vi "PB-01 Interface.vi"(6 "Device Inputs":dbl[](array[numeric]), 8 "error in":errorcluster, 9 "Device Outputs in":dbl[](array[numeric]), 10 "DCM Ref":refnum<class "DCM - RT.lvclass">, 11 "PB-01 in":T1={"FIFO Indexes"={"Write"={"Clear Faults"=0, "ESTTL Setup"=[], "UEGO Control"={"UEGO1Enable"=-1, "UEGO2Enable"=-1, "UEGO1Range"=-1, "UEGO2Range"=-1, "FilterCutoff (Hz)"=-1}}, "Read"={"UEGO Sensor Results"={"UEGO1Lambda"=-1, "UEGO1Phi"=-1, "UEGO1AFRatio"=-1, "UEGO1Ip (mA)"=-1, "UEGO2Lambda"=-1, "UEGO2Phi"=-1, "UEGO2AFRatio"=-1, "UEGO2Ip (mA)"=-1}, "UEGO Temperature (C)"={"UEGO1Temp (C)"=-1, "UEGO2Temp (C)"=-1, "UEGO1Hot"=-1, "UEGO2Hot"=-1}, "UEGO Diagnostics"={"UEGO1SensorFault"=-1, "UEGO2SensorFault"=-1, "UEGO1HeaterFault"=-1, "UEGO2HeaterFault"=-1, "UEGOFuseStatus"=-1, "Battery (V)"=-1, "LSUType"=-1}}}, "Settings"={"VR-Hall Mode Select"=[enum."VR Adaptive Arm", enum."VR Adaptive Arm", enum."VR Adaptive Arm", enum."VR Adaptive Arm", enum."VR Adaptive Arm"], "VR-Hall Arming Threshold [V]"=[0.0, 0.0, 0.0, 0.0, 0.0], "ESTTL Command Enabled"=FALSE}} {"FIFO Indexes"."Read"."UEGO Diagnostics"."LSUType" format="%02.0f"; "FIFO Indexes"."Read"."UEGO Diagnostics"."UEGOFuseStatus" format="%02.0f"}) -> (0 "error out":errorcluster, 1 "Device Outputs out":dbl[](array[numeric]), 2 "DCM Ref":refnum<class "DCM - RT.lvclass">, 3 "PB-01 out":T1={"FIFO Indexes"={"Write"={"Clear Faults"=0, "ESTTL Setup"=[], "UEGO Control"={"UEGO1Enable"=-1, "UEGO2Enable"=-1, "UEGO1Range"=-1, "UEGO2Range"=-1, "FilterCutoff (Hz)"=-1}}, "Read"={"UEGO Sensor Results"={"UEGO1Lambda"=-1, "UEGO1Phi"=-1, "UEGO1AFRatio"=-1, "UEGO1Ip (mA)"=-1, "UEGO2Lambda"=-1, "UEGO2Phi"=-1, "UEGO2AFRatio"=-1, "UEGO2Ip (mA)"=-1}, "UEGO Temperature (C)"={"UEGO1Temp (C)"=-1, "UEGO2Temp (C)"=-1, "UEGO1Hot"=-1, "UEGO2Hot"=-1}, "UEGO Diagnostics"={"UEGO1SensorFault"=-1, "UEGO2SensorFault"=-1, "UEGO1HeaterFault"=-1, "UEGO2HeaterFault"=-1, "UEGOFuseStatus"=-1, "Battery (V)"=-1, "LSUType"=-1}}}, "Settings"={"VR-Hall Mode Select"=[enum."VR Adaptive Arm", enum."VR Adaptive Arm", enum."VR Adaptive Arm", enum."VR Adaptive Arm", enum."VR Adaptive Arm"], "VR-Hall Arming Threshold [V]"=[0.0, 0.0, 0.0, 0.0, 0.0], "ESTTL Command Enabled"=FALSE}} {"FIFO Indexes"."Read"."UEGO Diagnostics"."LSUType" format="%02.0f"; "FIFO Indexes"."Read"."UEGO Diagnostics"."UEGOFuseStatus" format="%02.0f"})   [LabVIEW 2015]
uses:
  <vilib>/Powertrain Controls/Device Drivers/DCM/PB-01/RT/PB - 01 - RT.lvclass
  <vilib>/Powertrain Controls/Device Drivers/DCM/ESTTL/RT/DCM - RT - ESTTL.lvlib
  DCM-NIVS-RT/PB-01.ctl
  <vilib>/Powertrain Controls/Device Drivers/DCM/Rev0/RT/DCM - RT.lvclass
  <vilib>/Powertrain Controls/Device Drivers/VR-Hall/RevC/Real-Time/Support/Vr_Hall_mode_control_revc.ctl
  DCM-NIVS-RT/ESTTL Setup Indexes.ctl
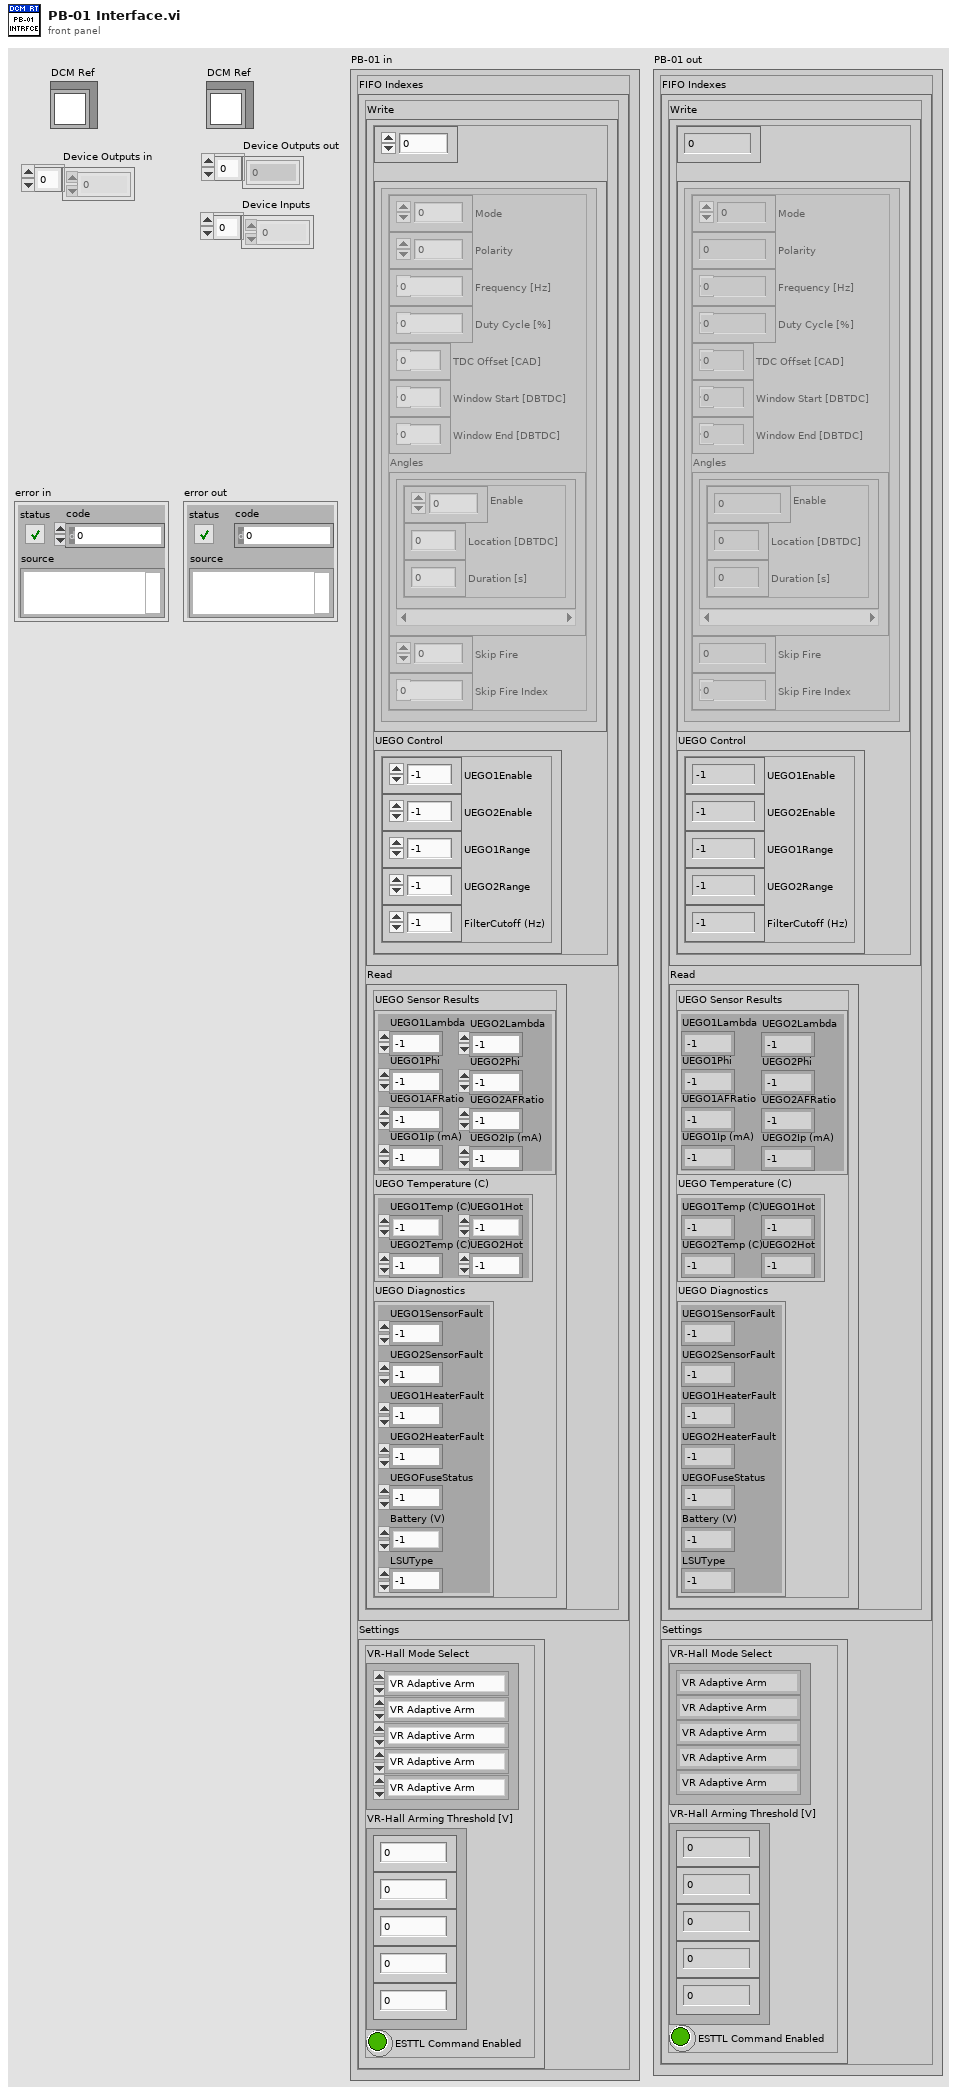
[diagram p1: front panel]
types:
  T1 = typedef "PB-01.ctl" = cluster{"FIFO Indexes":cluster{"Write":cluster{"Clear Faults":i32, "ESTTL Setup":T2[], "UEGO Control":cluster{"UEGO1Enable":i32, "UEGO2Enable":i32, "UEGO1Range":i32, "UEGO2Range":i32, "FilterCutoff (Hz)":i32}}, "Read":cluster{"UEGO Sensor Results":cluster{"UEGO1Lambda":i32, "UEGO1Phi":i32, "UEGO1AFRatio":i32, "UEGO1Ip (mA)":i32, "UEGO2Lambda":i32, "UEGO2Phi":i32, "UEGO2AFRatio":i32, "UEGO2Ip (mA)":i32}, "UEGO Temperature (C)":cluster{"UEGO1Temp (C)":i32, "UEGO2Temp (C)":i32, "UEGO1Hot":i32, "UEGO2Hot":i32}, "UEGO Diagnostics":cluster{"UEGO1SensorFault":i32, "UEGO2SensorFault":i32, "UEGO1HeaterFault":i32, "UEGO2HeaterFault":i32, "UEGOFuseStatus":i32, "Battery (V)":i32, "LSUType":i32}}}, "Settings":cluster{"VR-Hall Mode Select":T3[], "VR-Hall Arming Threshold [V]":dbl[], "ESTTL Command Enabled":bool}}
  T2 = typedef "ESTTL Setup Indexes.ctl" = cluster{"Mode":i32, "Polarity":i32, "Frequency [Hz]":i32, "Duty Cycle [%]":i32, "TDC Offset [CAD]":i32, "Window Start [DBTDC]":i32, "Window End [DBTDC]":i32, "Angles":cluster{"Enable":i32, "Location [DBTDC]":i32, "Duration [s]":i32}[], "Skip Fire":i32, "Skip Fire Index":i32}
  T3 = typedef "Vr_Hall_mode_control_revc.ctl" = enum32{"VR Adaptive Arm", "VR Manual Arm", "Hall", "Hall w/ Pull-up"}
  T4 = typedef "DCM - RT - ESTTL.lvlib/Setup.ctl" = cluster{"Mode":T5, "Polarity":bool, "Frequency [Hz]":sgl, "Duty Cycle [%]":sgl, "TDC Offset [CAD]":sgl, "Window Start [DBTDC]":sgl, "Window End [DBTDC]":sgl, "Angles":T6[], "Skip Fire":bool, "Skip Fire Index":u8}
  T5 = typedef "DCM - FPGA - ESTTL.lvlib/Mode.ctl" = enum8{"Off", "Pulse Width Modulation", "Engine Position Tracking"}
  T6 = typedef "DCM - RT - ESTTL.lvlib/Angle Control.ctl" = cluster{"Enable":bool, "Location [DBTDC]":sgl, "Duration [s]":sgl}
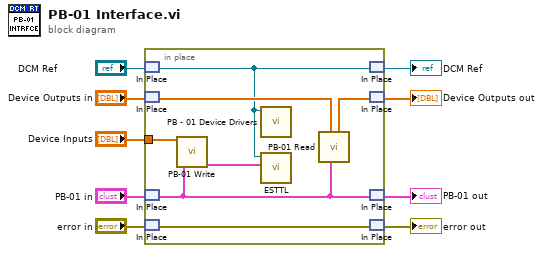
[diagram p0: block diagram]
diagram:
  n1 = in-place {
    in-place-border: "Device Inputs" -> [w15]
    n2 = in-place-match #1("DCM Ref") -> (w11:refnum<class "DCM - RT.lvclass">)
    n3 = in-place-match #2("Device Outputs in") -> (w14:dbl[])
    n4 = in-place-match #3("PB-01 in") -> (w10:T1)
    n5 = in-place-match #4("error in") -> (w16:errorcluster)
    n6 = call "PB-01 Write.vi"("Device Inputs"=w15, "PB-01 in"=w10) -> ("ESTTL Setup"=w12:T4[])  [unwired: 9 in, 4 out]
    n7 = call <vilib>:"PB - 01 Device Drivers.vi"("DCM Reference"=w11) -> ()  [unwired: 11 in]
    n8 = call <vilib>:"ESTTL.vi"("ESTTL Setup"=w12, "DCM Reference"=w11) -> ()  [unwired: 10 in]
    n9 = call "PB-01 Read.vi"("PB-01 in"=w10, "Device Outputs in"=w14) -> ("Device Outputs out"=w13:dbl[])  [unwired: 9 in]
    n10 = in-place-match #1(w11) -> (→"DCM Ref":refnum<class "DCM - RT.lvclass">)
    n11 = in-place-match #2(w13) -> (→"Device Outputs out":dbl[])
    n12 = in-place-match #3(w10) -> (→"PB-01 out":T1)
    n13 = in-place-match #4(w16) -> (→"error out":errorcluster)
  }
